vi "ReadFromFile.vi"(8 "operation (0:open)":T1(ring), 11 "file path (use dialog)":path) -> (0 "Open or create Control":string[][](table), 1 "Open Control":string[][](table), 2 "text 2":string, 3 "Array":string[][](array[string]))   [LabVIEW 2023]
panel:
  out "text":string
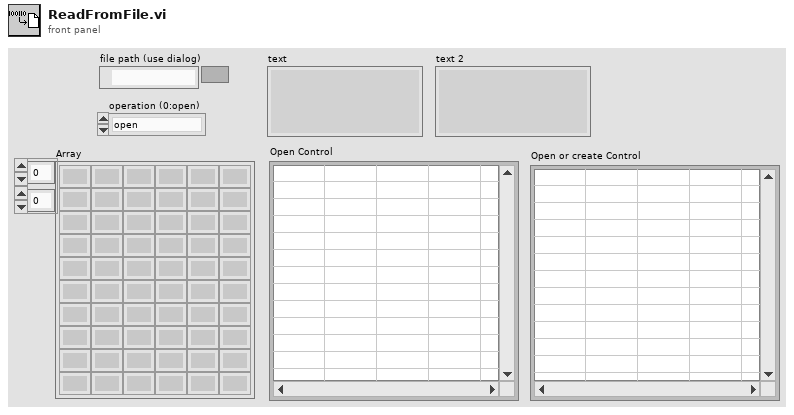
[diagram p1: front panel]
types:
  T1 = enum16{"open", "replace", "create", "open or create", "replace or create", "replace or create with confirmation"}
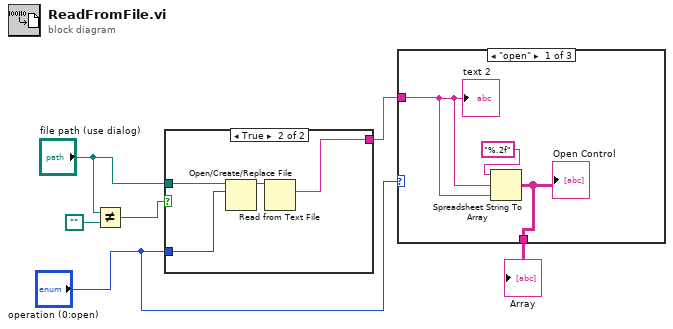
[diagram p0: block diagram]
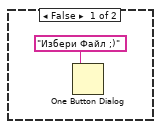
[diagram p2: hidden frame]
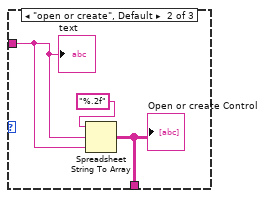
[diagram p3: hidden frame]
diagram:
  n1 = Not Equal?(x="file path (use dialog)", y=path "") -> (x != y?=w2:bool)
  n2 = case shown="True" w2 {
    tunnel: "file path (use dialog)" -> [_ w11]
    tunnel: [_ w9] -> w6
    tunnel: "operation (0:open)" -> [_ w8]
    frame False {
      n3 = One Button Dialog(message="Избери Файл ;)") -> ()  [unwired: 1 in, 1 out]
    }
    frame True {
      n4 = Open/Create/Replace File(file path (use dialog)=w11, operation (0:open)=w8) -> (refnum out=w10:refnum<file>)  [unwired: 4 in, 2 out]
      n5 = Read from Text File(file (use dialog)=w10) -> (text=w9:string)  [unwired: 3 in, 3 out]
    }
  }
  n6 = case shown="\"open\"" "operation (0:open)" {
    tunnel: w6 -> [w13 w16 _]
    tunnel: [w12 w15 _] -> w1
    frame "open" {
      n7 = Spreadsheet String To Array(format string="%.2f", spreadsheet string=w13, array type (2D Dbl)=w13) -> (array=w12:string[][])  [unwired: 1 in]
      "Open Control" <- w12
      "text 2" <- w13
    }
    frame "open or create", Default {
      n8 = Spreadsheet String To Array(format string="%.2f", spreadsheet string=w16, array type (2D Dbl)=w16) -> (array=w15:string[][])  [unwired: 1 in]
      "Open or create Control" <- w15
      "text" <- w16
    }
    frame "replace" {
    }
  }
  "Array" <- w1
